vi "Scott -- strain -- voltage-wave-form-generator-test.vi"() -> ()   [LabVIEW 2014]
uses:
  voltage-wave-generator-parameters.ctl
  votage-control.ctl
panel:
  in  "voltage-parameters-IN":T1
  out "XY Graph":cluster{dbl[], dbl[]}(graph)
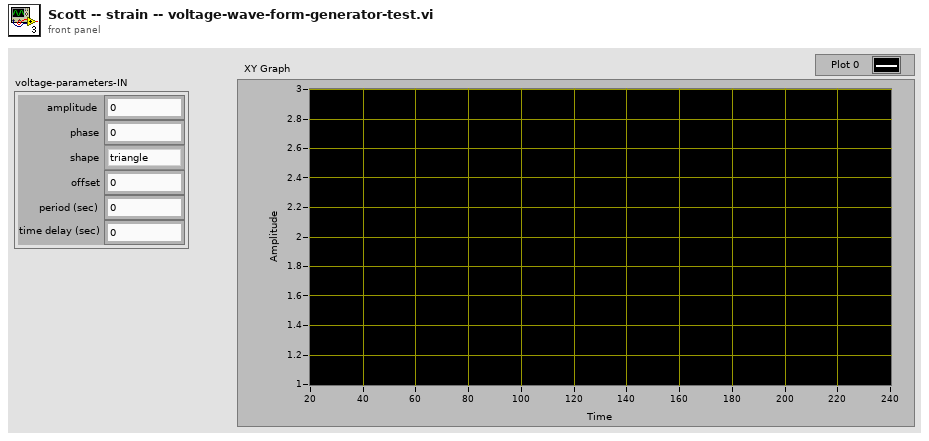
[diagram p1: front panel]
types:
  T1 = typedef "voltage-wave-generator-parameters.ctl" = cluster{"amplitude":dbl, "phase":dbl, "shape":enum16{"triangle"}, "offset":dbl, "period (sec)":dbl, "time delay (sec)":dbl}
  T2 = typedef "votage-control.ctl" = enum16{"reset", "next"}
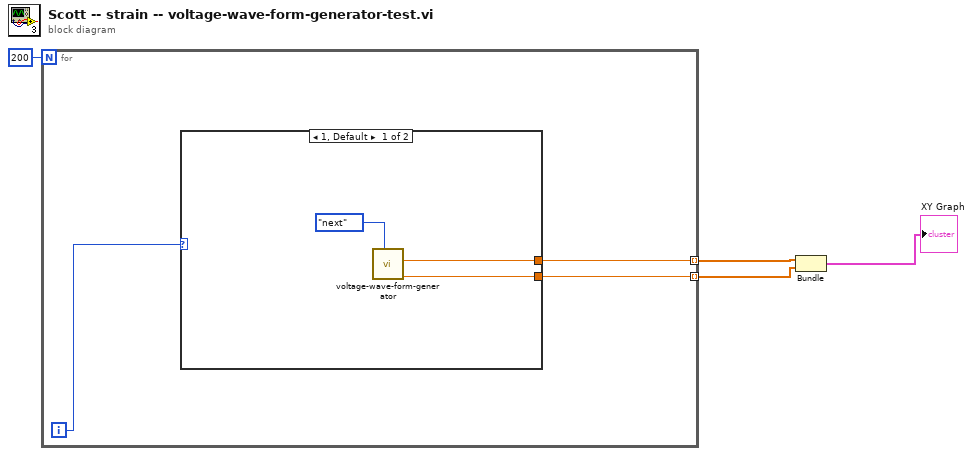
[diagram p0: block diagram]
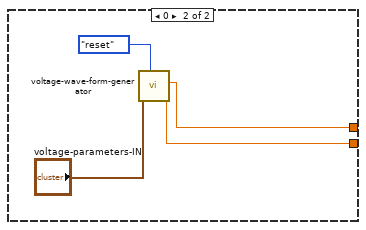
[diagram p2: hidden frame]
diagram:
  n1 = for {
    N: 200 -> [_]
    tunnel: [w6] -> w4 mode=indexing
    tunnel: [w5] -> w3 mode=indexing
    i -> [w7]
    n2 = case shown="1, Default" w7 {
      tunnel: [w9 w12] -> w6
      tunnel: [w8 w11] -> w5
      frame 1, Default {
        n3 = call "voltage-wave-form-generator.vi"("voltage-wave-control"=votage-control."next") -> ("voltage out (V)"=w8:dbl, "time (sec) out"=w9:dbl)  [unwired: 8 in, 1 out]
      }
      frame 0 {
        n4 = call "voltage-wave-form-generator.vi"("voltage-wave-control"=votage-control."reset", "voltage-parameters-IN"="voltage-parameters-IN") -> ("voltage out (V)"=w11:dbl, "time (sec) out"=w12:dbl)  [unwired: 7 in, 1 out]
      }
    }
  }
  n5 = Bundle(w4, w3) -> (→"XY Graph":cluster{dbl[], dbl[]})  [unwired: 1 in]
